vi "Average Measure (More) than one.vi"(0 "VISA resource name":refnum<visa-resource-name>, 1 "Measurement Function (0: Rise Time)":i32(ring) items=["Rise Time", "Fall Time", "Frequency", "Period", "Voltage RMS(AC)", "Voltage RMS(DC)", "Voltage RMS (AC,cycle)", "Voltage RMS (DC,cycle)", "Voltage Max", "Voltage Min", "Voltage Middle", "Voltage Vpp", "Voltage High", "Voltage Low", "Voltage Average", "Voltage Average (cycle)", "Width Negative", "Width Positive", "Duty Cycle Positive", "Amplitude", "Overshoot", "Preshoot", "Voltage Base", "Voltage Upper", "Time Max", "Time Min", "Color Grade Crossing", "Color Grade Eye Width", "Color Grade Eye Height", "Color Grade Eye Q-Factory", "Color Grade Eye Duty Cycle Distortion(Percent)", "Color Grade Eye Duty Cycle Distortion(Time)", "Color Grade Eye Jitter(PP)", "Color Grade Eye Width(RMS)", "Cycle-cycle Duty Jitter(Rising)", "Cycle-cycle Duty Jitter(Falling)", "Cycle-cycle Jitter(Rising)", "Cycle-cycle Jitter(Falling)", "Cycle-cycle - Width", "Cycle-cycle + Width", "Date Rate", "Unit Interval", "FFT Delta Frequency", "FFT Delta Magnitude", "FFT Frequency", "FFT Magnitude", "Slew Rate", "Area (Entire Display)", "Area(Single Cycle)", "Duty Cycle (Rising)", "Duty Cycle (Falling)"], 2 "Averages":u32=32, 5 "Channel (1: Channel 1)":i32(ring)=1 items=["Channel 1"=1, "Channel 2"=2, "Channel 3"=3, "Channel 4"=4, "Function 1"=5, "Function 2"=6, "Function 3"=7, "Function 4"=8, "Memory 1"=9, "Memory 2"=10, "Memory 3"=11, "Memory 4"=12], 7 "Maximum Time (10000ms)":u32=10000, 9 "Channel (1: Channel 1) 2":i32(ring)=5 items=["Channel 1"=1, "Channel 2"=2, "Channel 3"=3, "Channel 4"=4, "Function 1"=5, "Function 2"=6, "Function 3"=7, "Function 4"=8, "Memory 1"=9, "Memory 2"=10, "Memory 3"=11, "Memory 4"=12], 11 "error in (no error)":errorcluster, 12 "Measurement Function (0: Rise Time) 2":i32(ring)=17 items=["Rise Time", "Fall Time", "Frequency", "Period", "Voltage RMS(AC)", "Voltage RMS(DC)", "Voltage RMS (AC,cycle)", "Voltage RMS (DC,cycle)", "Voltage Max", "Voltage Min", "Voltage Middle", "Voltage Vpp", "Voltage High", "Voltage Low", "Voltage Average", "Voltage Average (cycle)", "Width Negative", "Width Positive", "Duty Cycle Positive", "Amplitude", "Overshoot", "Preshoot", "Voltage Base", "Voltage Upper", "Time Max", "Time Min", "Color Grade Crossing", "Color Grade Eye Width", "Color Grade Eye Height", "Color Grade Eye Q-Factory", "Color Grade Eye Duty Cycle Distortion(Percent)", "Color Grade Eye Duty Cycle Distortion(Time)", "Color Grade Eye Jitter(PP)", "Color Grade Eye Width(RMS)", "Cycle-cycle Duty Jitter(Rising)", "Cycle-cycle Duty Jitter(Falling)", "Cycle-cycle Jitter(Rising)", "Cycle-cycle Jitter(Falling)", "Cycle-cycle - Width", "Cycle-cycle + Width", "Date Rate", "Unit Interval", "FFT Delta Frequency", "FFT Delta Magnitude", "FFT Frequency", "FFT Magnitude", "Slew Rate", "Area (Entire Display)", "Area(Single Cycle)", "Duty Cycle (Rising)", "Duty Cycle (Falling)"], 13 "Max Errors":u32=40) -> (4 "VISA resource name out":refnum<visa-resource-name>, 8 "measurements":dbl[](array[numeric]), 15 "error out":errorcluster)   [LabVIEW 2009]
uses:
  <vilib>/Analysis/NI_AALBase.lvlib
panel:
  out "Measure Error 5":dbl caption="Measurement"
  out "Measure Average 5":dbl caption="Measurement"
  out "Measure Error 4":dbl caption="Measurement"
  out "Measure Average 4":dbl caption="Measurement"
  out "Measure Error 3":dbl caption="Measurement"
  out "Measure Average 3":dbl caption="Measurement"
  out "Measure Error 2":dbl caption="Measurement"
  out "Measure Average 2":dbl caption="Measurement"
  out "Measure Error":dbl caption="Measurement"
  out "Measure Average":dbl caption="Measurement"
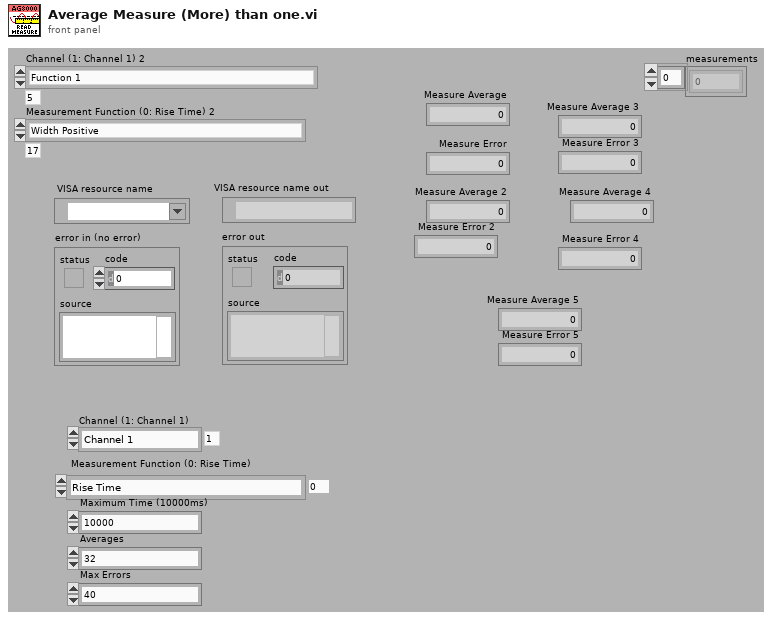
[diagram p1: front panel]
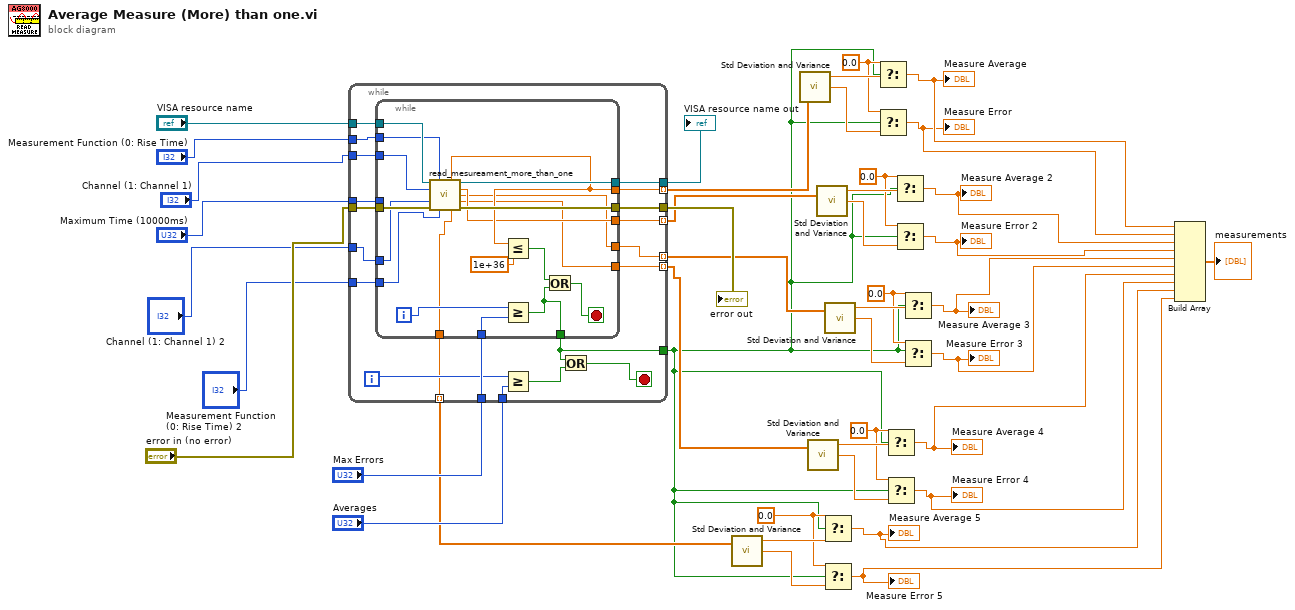
[diagram p0: block diagram]
diagram:
  w16 = 0.0 ("t")
  w22 = 0.0 ("t")
  w25 = 0.0 ("t")
  w28 = 0.0 ("t")
  w31 = 0.0 ("t")
  n1 = while {
    tunnel: "VISA resource name" -> [w63]
    tunnel: "Channel (1: Channel 1)" -> [w50]
    tunnel: "Measurement Function (0: Rise Time)" -> [w62]
    tunnel: "Maximum Time (10000ms)" -> [w61]
    tunnel: "error in (no error)" -> [w60]
    tunnel: [w59] -> w38
    tunnel: [w58] -> w34 mode=indexing
    tunnel: [w57] -> w37
    tunnel: "Max Errors" -> [w56]
    tunnel: "Averages" -> [w54]
    tunnel: [w51] -> w12
    tunnel: [w49] -> w21 mode=indexing
    tunnel: [w48] -> w20 mode=indexing
    tunnel: [w47] -> w19 mode=indexing
    tunnel: [w46] -> w13 mode=indexing
    tunnel: "Channel (1: Channel 1) 2" -> [w45]
    tunnel: "Measurement Function (0: Rise Time) 2" -> [w44]
    i -> [w55]
    stop <- w52 stop-if-true
    n2 = while {
      tunnel: w63 -> [w73]
      tunnel: w62 -> [w64]
      tunnel: w61 -> [_]
      tunnel: w60 -> [w74]
      tunnel: [w75] -> w59
      tunnel: [w72] -> w58
      tunnel: [w76] -> w57
      tunnel: w56 -> [w79]
      tunnel: [w77] -> w51
      tunnel: w50 -> [w65]
      tunnel: [w71] -> w49
      tunnel: [w70] -> w48
      tunnel: [w69] -> w47
      tunnel: [w68] -> w46
      tunnel: w45 -> [w66]
      tunnel: w44 -> [w67]
      i -> [w80]
      stop <- w78 stop-if-true
      n3 = call "read_mesureament_more_than_one.vi"("VISA resource name"=w73, "Measurement Function (0: Rise Time)"=w64, "Channel (1: Channel 1)"=w65, "Channel (1: Channel 1) 2"=w66, "error in (no error)"=w74, "Measurement Function (0: Rise Time) 2"=w67) -> ("Measurement"=w72:dbl, "VISA resource name out"=w76:refnum<visa-resource-name>, "Measurement 2"=w71:dbl, "Measurement 3"=w70:dbl, "Measurement 4"=w69:dbl, "Delta Time(s)"=w68:dbl, "error out"=w75:errorcluster)  [unwired: 3 in]
      n4 = Less Or Equal?(x=w72, y=1e+36) -> (x <= y?=w82:bool)
      n5 = Greater Or Equal?(x=w80, y=w79) -> (x >= y?=w77:bool)
      n6 = Or(x=w82, y=w77) -> (x .or. y?=w78:bool)
    }
    n7 = Greater Or Equal?(x=w55, y=w54) -> (x >= y?=w53:bool)
    n8 = Or(x=w51, y=w53) -> (x .or. y?=w52:bool)
  }
  "error out" <- w38
  "VISA resource name out" <- w37
  n9 = call <vilib>:"Std Deviation and Variance.vi"("X"=w13) -> ("mean"=w17:dbl, "standard deviation"=w18:dbl)  [unwired: 1 in, 1 out]
  n10 = call <vilib>:"Std Deviation and Variance.vi"("X"=w34) -> ("mean"=w32:dbl, "standard deviation"=w33:dbl)  [unwired: 1 in, 1 out]
  n11 = call <vilib>:"Std Deviation and Variance.vi"("X"=w19) -> ("mean"=w23:dbl, "standard deviation"=w24:dbl)  [unwired: 1 in, 1 out]
  n12 = call <vilib>:"Std Deviation and Variance.vi"("X"=w21) -> ("mean"=w29:dbl, "standard deviation"=w30:dbl)  [unwired: 1 in, 1 out]
  n13 = Select(t=w16, s=w12, f=w17) -> (s? t:f=w3:dbl)
  "Measure Average 5" <- w3
  n14 = Select(t=w16, s=w12, f=w18) -> (s? t:f=w2:dbl)
  "Measure Error 5" <- w2
  n15 = call <vilib>:"Std Deviation and Variance.vi"("X"=w20) -> ("mean"=w26:dbl, "standard deviation"=w27:dbl)  [unwired: 1 in, 1 out]
  n16 = Select(t=w31, s=w12, f=w32) -> (s? t:f=w11:dbl)
  "Measure Average" <- w11
  n17 = Select(t=w31, s=w12, f=w33) -> (s? t:f=w10:dbl)
  "Measure Error" <- w10
  n18 = Select(t=w22, s=w12, f=w23) -> (s? t:f=w5:dbl)
  "Measure Average 4" <- w5
  n19 = Select(t=w22, s=w12, f=w24) -> (s? t:f=w4:dbl)
  "Measure Error 4" <- w4
  n20 = Select(t=w28, s=w12, f=w29) -> (s? t:f=w9:dbl)
  "Measure Average 2" <- w9
  n21 = Select(t=w28, s=w12, f=w30) -> (s? t:f=w8:dbl)
  "Measure Error 2" <- w8
  n22 = Select(t=w25, s=w12, f=w26) -> (s? t:f=w7:dbl)
  "Measure Average 3" <- w7
  n23 = Select(t=w25, s=w12, f=w27) -> (s? t:f=w6:dbl)
  "Measure Error 3" <- w6
  n24 = Build Array(w11, w10, w9, w8, w7, w6, w5, w4, w3, w2) -> (→"measurements":dbl[])
